vi "fpga_Timestamps_writer_32bit.vi"(1 "All Ch Timestamps":T1={"Timestamp"=0, "Data available"=TRUE}) -> ()   [LabVIEW 2011]
uses:
  Time Stamp Data.ctl
  <vilib>/rvi/interface/RandomDataEmulation/niFpgaRandomDataHandleErrors.vi
  <vilib>/rvi/interface/RandomDataEmulation/nirviRandomDataFPGAFIFO.vi
  <vilib>/rvi/DataTransferAndStorage/Container/XNode/niFpgaContainer.xnode
  <vilib>/rvi/interface/RandomDataEmulation/nirviRandomDataFpgaReadWriteTemplate.vi
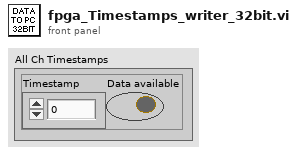
[diagram p1: front panel]
types:
  T1 = typedef "Time Stamp Data.ctl" = cluster{"Timestamp":u32, "Data available":bool}
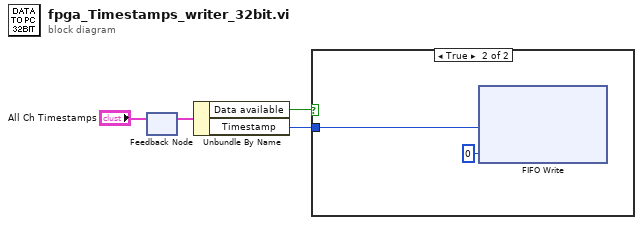
[diagram p0: block diagram]
diagram:
  n1 = feedback-in #1("All Ch Timestamps") -> ()
  n2 = feedback #1() -> (w1:T1)  [unwired: 1 in]
  n3 = Unbundle By Name(w1) -> ("Data available"=w3:bool, "Timestamp"=w2:u32)
  n4 = case shown="True" w3 {
    tunnel: w2 -> [_ w5]
    frame False {
    }
    frame True {
      n5 = xnode ("FIFO Write")("Element"=w5, "Timeout"=0) -> ()  [unwired: 1 in, 2 out]
    }
  }
